vi "liblinear_add_problem_padding.vi"(8 "error in (no error)":errorcluster, 11 "problem":T3={"y"=[], "x"=[], "bias"=-1.0}) -> (0 "error out":errorcluster, 3 "problem padded":T1={"y"=[], "x"=[], "bias"=-1.0})   [LabVIEW 2014]
uses:
  Controls/liblinear_problem.ctl
  Libsvm Wrapper/Controls/svm_node.ctl
  Controls/liblinear_problem_padded.ctl
  Controls/liblinear_node_padded.ctl
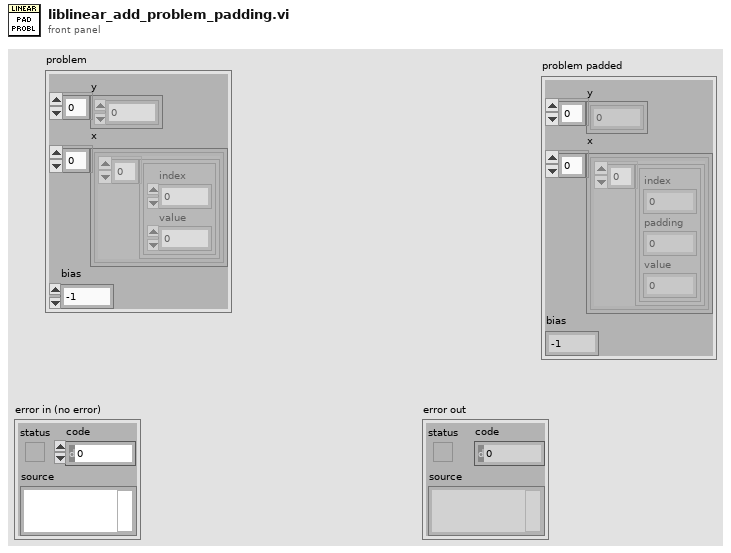
[diagram p1: front panel]
types:
  T1 = typedef "liblinear_problem_padded.ctl" = cluster{"y":dbl[], "x":cluster{T2[]}[], "bias":dbl}
  T2 = typedef "liblinear_node_padded.ctl" = cluster{"index":i32, "padding":i32, "value":dbl}
  T3 = typedef "liblinear_problem.ctl" = cluster{"y":dbl[], "x":cluster{T4[]}[], "bias":dbl}
  T4 = typedef "svm_node.ctl" = cluster{"index":i32, "value":dbl}
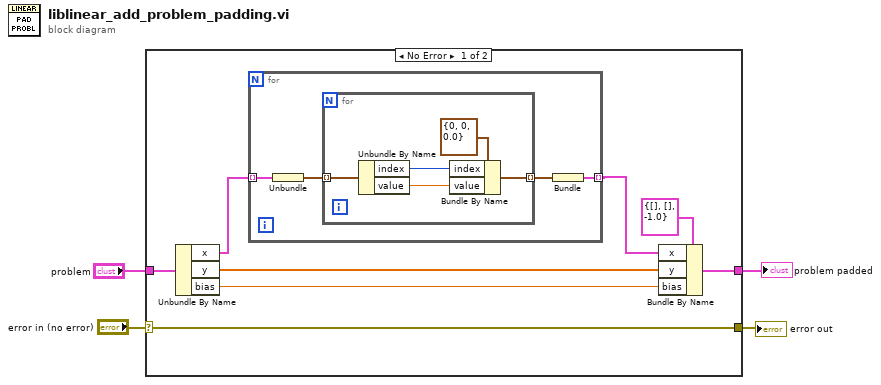
[diagram p0: block diagram]
diagram:
  n1 = case shown="No Error" "error in (no error)" {
    selector: "error in (no error)" -> [w7 w22]
    tunnel: [w7 w22] -> w4
    tunnel: "problem" -> [w11 _]
    tunnel: [w8 _] -> w1
    frame No Error {
      n2 = Unbundle By Name(w11) -> ("x"=w12:cluster{T4[]}[], "y"=w9:dbl[], "bias"=w5:dbl)
      n3 = for {
        tunnel: w12 -> [w16] mode=indexing
        tunnel: [w13] -> w10 mode=indexing
        n4 = Unbundle(w16) -> (w15:T4[])
        n5 = for {
          tunnel: w15 -> [w21] mode=indexing
          tunnel: [w18] -> w14 mode=indexing
          n6 = Unbundle By Name(w21) -> ("index"=w20:i32, "value"=w19:dbl)
          n7 = Bundle By Name(cluster=T2 {"index"=0, "padding"=0, "value"=0.0} ("feature_node"), "index"=w20, "value"=w19) -> (w18:T2)
        }
        n8 = Bundle(w14) -> (w13:cluster{T2[]})  [unwired: 1 in]
      }
      n9 = Bundle By Name(cluster=T1 {"y"=[], "x"=[], "bias"=-1.0} ("problem padded"), "x"=w10, "y"=w9, "bias"=w5) -> (w8:T1)
    }
    frame Error {
    }
  }
  "error out" <- w4
  "problem padded" <- w1
